vi "Read from HR DB.vi"(8 "error in (no error)":errorcluster, 9 "Length (-1)":i32=-1, 10 "Modbus Address":u16, 11 "MB Data Block in":refnum<class "MB Data Block.lvclass">) -> (0 "error out":errorcluster, 2 "Data out":u16[](array[numeric]), 3 "MB Data Block out":refnum<class "MB Data Block.lvclass">)   [LabVIEW 2018, in "MB PLC Client.lvlib" / "MB Data Block.lvclass"]
uses:
  MB Data Block.lvclass
  MB Data Block.lvclass/MB Data Block.ctl
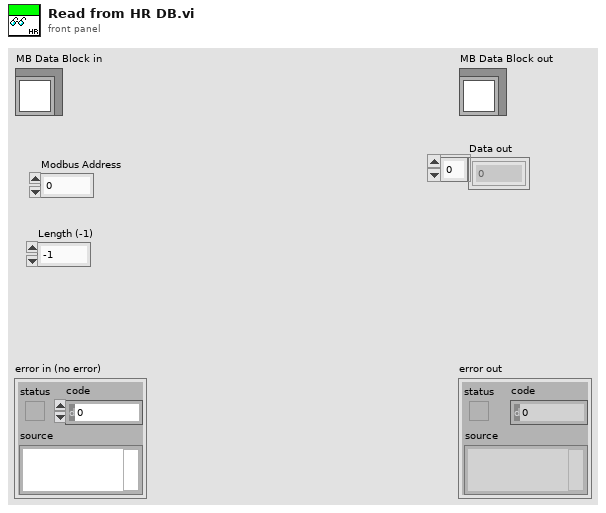
[diagram p1: front panel]
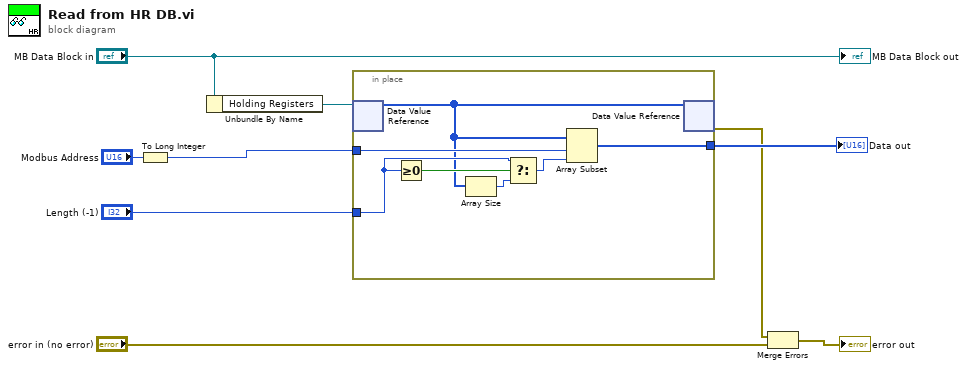
[diagram p0: block diagram]
diagram:
  n1 = To Long Integer(number="Modbus Address") -> (32bit integer=w8:i32)
  n2 = Unbundle By Name("MB Data Block in") -> ("Holding Registers"=w5:refnum<data-value>)
  n3 = in-place {
    in-place-border: w8 -> [w16]
    in-place-border: "Length (-1)" -> [w15]
    in-place-border: [w14] -> w6
    n4 = in-place-dvr #1(w5) -> (w10:u16[])  [unwired: 1 out]
    n5 = Greater Or Equal To 0?(x=w15) -> (x >= 0?=w12:bool)
    n6 = Array Size(array=w10) -> (size(s)=w13:i32)
    n7 = Select(t=w15, s=w12, f=w13) -> (s? t:f=w11:i32)
    n8 = Array Subset(array=w10, index=w16, length=w11) -> (w14:u16[])
    n9 = in-place-dvr #1(w10) -> (w3:errorcluster)  [unwired: 1 out]
  }
  "Data out" <- w6
  n10 = Merge Errors(w3, "error in (no error)") -> (→"error out":errorcluster)
  "MB Data Block out" <- "MB Data Block in"
